vi "MP3音乐播放器.vi"(0 "歌曲文件夹":path) -> (7 "播放列表":string[][](array[string]))   [LabVIEW 2014]
uses:
  <vilib>/Utility/inputDevices.llb/mouseAcquire.vi
panel:
  in  "WindowsMediaPlayer":refnum<k7>(container)
  out "当前播放：":string
  # "小林子音乐播放器"
  # "ps：如果大家觉得好就微信扫一扫右上角的二维码哦，加关注，小编每天都会更新不一样的 labview程序源码，和大家分享，共同进步！让你躺着也能学labview。。。（在微信添加好友 lablover也可以关注的）"
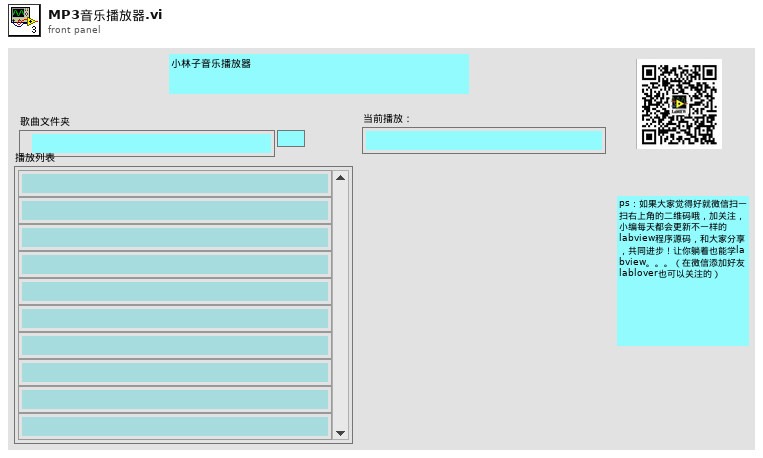
[diagram p1: front panel]
types:
  T1 = typedef "LVPositionTypeDef.ctl" = cluster{"Left":i32, "Top":i32}
  T2 = cluster{"button 1":bool, "button 2":bool, "button 3":bool, "button 4":bool}
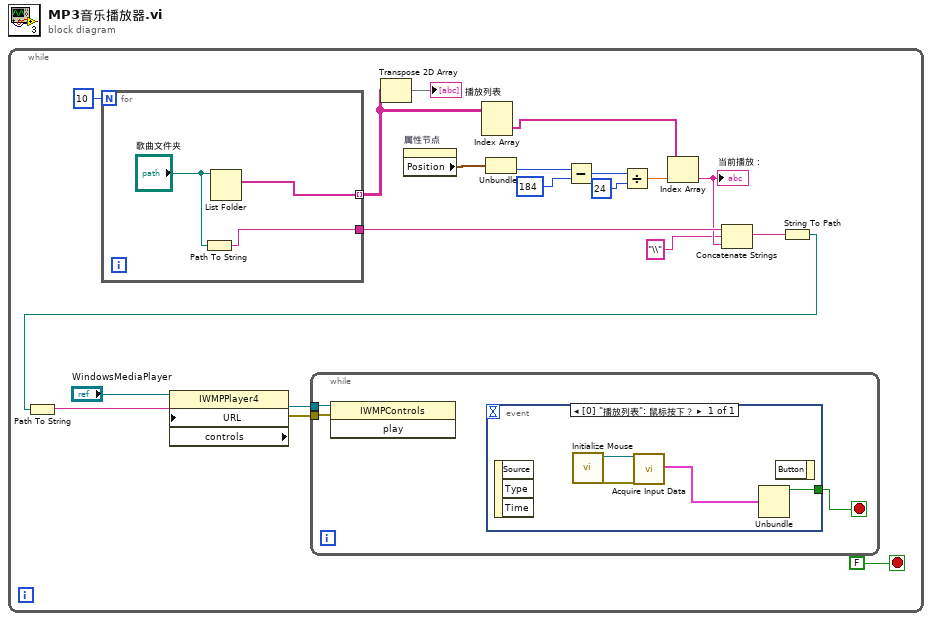
[diagram p0: block diagram]
diagram:
  n1 = while {
    stop <- FALSE stop-if-true
    n2 = for {
      N: 10 -> [_]
      tunnel: [w30] -> w18 mode=indexing
      tunnel: [w28] -> w10
      n3 = Path To String(path="歌曲文件夹") -> (string=w28:string)
      n4 = List Folder(path="歌曲文件夹") -> (filenames=w30:string[])  [unwired: 3 in, 3 out]
    }
    n5 = Transpose 2D Array(2D array=w18) -> (transposed array=→"播放列表":string[][])
    n6 = property on="属性节点" class="Str"() -> ("Position"=w16:T1)  [unwired: 2 in, 2 out]
    n7 = Index Array(array=w18) -> (element=w17:string[])  [unwired: 2 in]
    n8 = Unbundle(w16) -> ("Top"=w11:i32)  [unwired: 1 out]
    n9 = Subtract(x=w11, y=184) -> (x-y=w14:i32)
    n10 = Divide(x=w14, y=24) -> (x/y=w12:dbl)
    n11 = Index Array(array=w17, index=w12) -> (element=w9:string)
    "当前播放：" <- w9
    n12 = Concatenate Strings(w10, "\\" ("字符串"), w9) -> (w7:string)
    n13 = String To Path(string=w7) -> (path=w2:path)
    n14 = Path To String(path=w2) -> (string=w6:string)
    n15 = property on="属性节点" class="IWMPPlayer4"(reference="WindowsMediaPlayer", "URL"=w6) -> (error out=w4:errorcluster, "controls"=w5:refnum<k7>)  [unwired: 1 in, 1 out]
    n16 = while {
      tunnel: w5 -> [w23]
      tunnel: w4 -> [w22]
      stop <- w21 stop-if-true
      n17 = invoke class="IWMPControls" method="play"(reference=w23, error in=w22) -> ()  [unwired: 1 in, 3 out]
      n18 = event shown="[0] \"播放列表\": 鼠标按下？" {
        selector: _ -> [_]
        dyn-events: _ -> [_]
        timeout: _ -> [_]
        tunnel: [w24] -> w21
        event "播放列表": Mouse Down? {
          n19 = event-data() -> ()  [unwired: 1 in, 3 out]
          n20 = call <vilib>:"Initialize Mouse.vi"() -> ("error out"=w26:errorcluster, "device ID"=w27:refnum<k1>)  [unwired: 10 in]
          n21 = call-poly <vilib>:"Acquire Input Data.vi"("device ID"=w27, "error in (no error)"=w26) -> ("button info"=w25:T2)  [unwired: 14 in, 3 out]
          n22 = Unbundle(w25) -> ("button 1"=w24:bool)  [unwired: 3 out]
          n23 = event-data() -> ()  [unwired: 2 in, 1 out]
        }
      }
    }
  }
